vi "readPOS_ACT.vi"() -> ()   [LabVIEW 2015]
uses:
  <vilib>/Platform/TimedLoop/XDataNode/timing_clust.ctl
  <vilib>/Platform/TimedLoop/XDataNode/nitl_modes.ctl
  <vilib>/Platform/TimedLoop/XDataNode/wakeup.ctl
  <vilib>/Platform/TimedLoop/XDataNode/XDataNode.xnode
  <vilib>/Platform/TimedLoop/XDataNode/XDNodeRunTimeDep.lvlib
  <vilib>/ptbypt/NI_PtbyPt.lvlib
  labOpenShowVar.lvlib
panel:
  in  "周期":i64=100
  out "测量时间":u32
  in  "sample length":i32=100
  in  "initialize":bool caption="初始化"
  out "XY图":T1(graph)
  out "Z":dbl format="%.2f"
  out "Y":dbl format="%.2f"
  out "X":dbl format="%.2f"
  out "data":string
  in  "var":string="$POS_ACT"
  in  "停止":bool
  in  "地址":string="172.31.1.147"
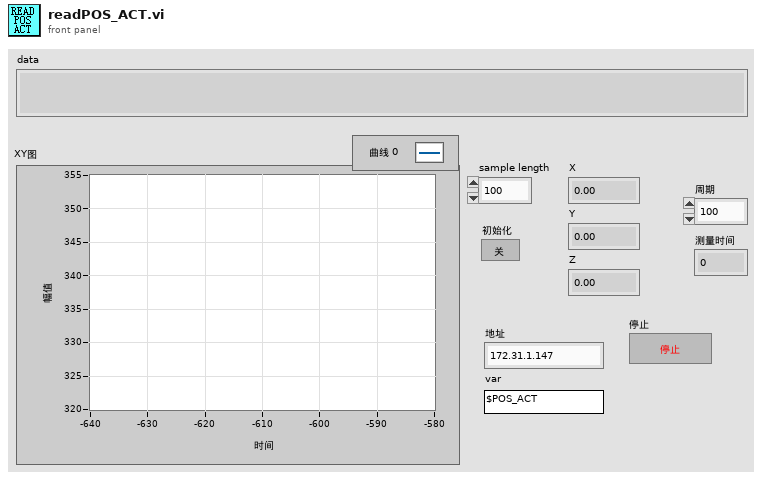
[diagram p1: front panel]
types:
  T1 = cluster{"Current Queue":dbl[], "Current Queue":dbl[]}
  T2 = typedef "XDNodeRunTimeDep.lvlib/timing_clust.ctl" = cluster{"Expected End [f-1]":u64, "Actual End [f-1]":u64, "Finished Late? [f-1]":bool, "Expected End [i-1]":u64, "Actual End [i-1]":u64, "Finished Late? [i-1]":bool, "Expected Start [i]":u64, "Actual Start [i]":u64, "Expected Start [f]":u64, "Actual Start [f]":u64, "Source Name":string, "Structure Name":string, "Period":i64, "Deadline":i64, "Offset":i64, "Start":i64, "Priority":i32, "Timeout":i32, "Mode":T3, "Wakeup Reason":T4, "Error":errorcluster, "Source Type":string, "Secondary Source Type":string, "Global End Time":u64, "Global Start Time":u64, "Frame Duration":u64, "Iteration Duration":u64, "Assigned CPU":i32, "I/O Scan Engine Mode":u32}
  T3 = typedef "XDNodeRunTimeDep.lvlib/nitl_modes.ctl" = enum32{"No Change", "Process missed periods, maintain original phase", "Discard missed periods, maintain original phase", "Process missed periods, ignore original phase", "Discard missed periods, ignore original phase"}
  T4 = typedef "XDNodeRunTimeDep.lvlib/wakeup.ctl" = enum32{"Normal", "Aborted", "Asynchronous wakeup", "Timing source error", "Timed loop error", "Timeout"}
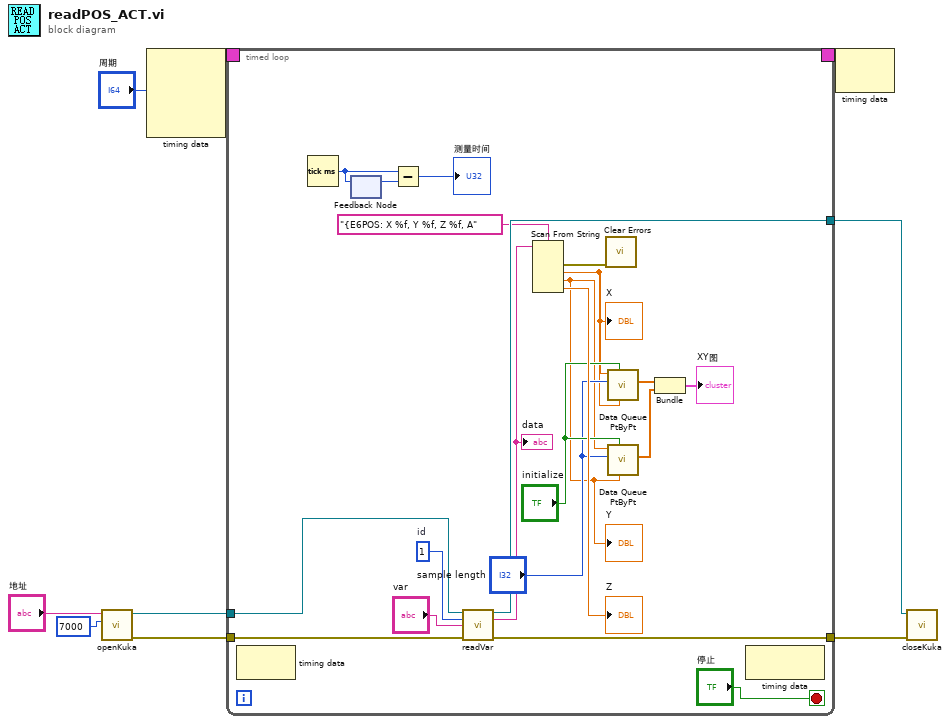
[diagram p0: block diagram]
diagram:
  n1 = call "openKuka.vi"("远程端口或服务名称"=u16 7000, "地址"="地址") -> ("错误输出"=w6:errorcluster, "TCP网络连接输出"=w7:refnum<k5>)  [unwired: 8 in]
  n2 = node-c288("周期") -> (w5:T2)  [unwired: 3 in]
  n3 = timed-loop {
    tunnel: w7 -> [w29]
    tunnel: w6 -> [w26]
    tunnel: [w25] -> w2
    tunnel: [w24] -> w3
    timing: w5 -> [_]
    timing-out: [_] -> w4
    stop <- "停止" stop-if-true
    w28 = u16 1  # id
    n4 = node-c288() -> ()  [unwired: 1 in, 1 out]
    n5 = Tick Count (ms)() -> (millisecond timer value=w12:u32)
    n6 = feedback-in #1(w12) -> ()
    n7 = feedback #1() -> (w11:u32)  [unwired: 1 in]
    n8 = Subtract(x=w12, y=w11) -> (x-y=→"测量时间":u32)
    n9 = call "readVar.vi"("TCP网络连接输入"=w29, "id"=w28, "var"="var", "错误输入（无错误）"=w26) -> ("TCP网络连接输出"=w24:refnum<k5>, "data out"=w23:string, "错误输出"=w25:errorcluster)  [unwired: 9 in]
    "data" <- w23
    n10 = Scan From String(format string="{E6POS: X %f, Y %f, Z %f, A" ("格式字符串"), input string=w23) -> (error out=w21:errorcluster, output 1=w17:dbl, output 2=w16:dbl, output 3=→"Z":dbl)  [unwired: 5 in, 2 out]
    "X" <- w17
    "Y" <- w16
    n11 = call <vilib>:"Clear Errors.vi"("error in (no error)"=w21) -> ()  [unwired: 5 in, 2 out]
    n12 = call <vilib>:"Data Queue PtByPt.vi"("initial queue element"=w17, "initialize"="initialize", "sample length"="sample length", "input data point"=w17) -> ("Current Queue"=w15:dbl[])  [unwired: 3 in, 4 out]
    n13 = call <vilib>:"Data Queue PtByPt.vi"("initial queue element"=w16, "initialize"="initialize", "sample length"="sample length", "input data point"=w16) -> ("Current Queue"=w14:dbl[])  [unwired: 3 in, 4 out]
    n14 = Bundle("Current Queue"=w15, "Current Queue"=w14) -> (→"XY图":T1)  [unwired: 1 in]
    n15 = node-c288() -> ()  [unwired: 1 in, 1 out]
  }
  n16 = node-c288(w4) -> ()  [unwired: 1 out]
  n17 = call "closeKuka.vi"("错误输入（无错误）"=w2, "TCP网络连接输入"=w3) -> ()  [unwired: 10 in]
